vi "Zmienne funkcjonalne.vi"() -> ()   [LabVIEW 2020]
uses:
  Control 4.ctl
panel:
  out "XY Graph":cluster{"Array 2":dbl[], "Array 2":dbl[]}(graph)
  in  "Enum":T1
  out "Array":dbl[][](array[numeric])
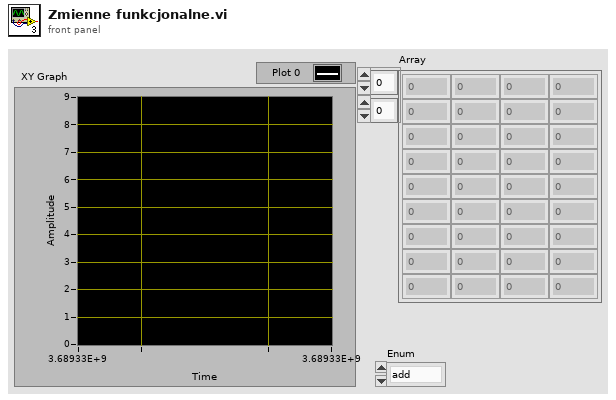
[diagram p1: front panel]
types:
  T1 = typedef "Control 4.ctl" = enum16{"add", "read", "readAll", "reset", "zapis_do_pliku", "odczyt_z_pliku"}
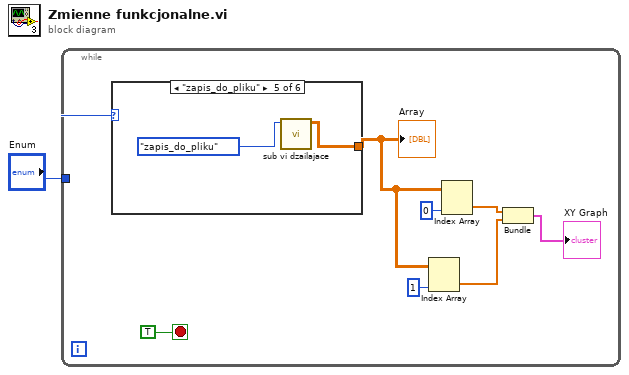
[diagram p0: block diagram]
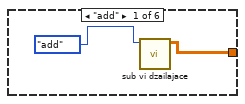
[diagram p2: hidden frame]
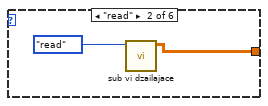
[diagram p3: hidden frame]
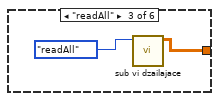
[diagram p4: hidden frame]
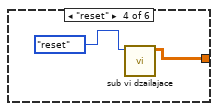
[diagram p5: hidden frame]
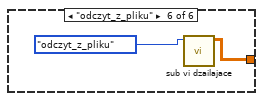
[diagram p6: hidden frame]
diagram:
  n1 = while {
    tunnel: "Enum" -> [w8]
    stop <- TRUE stop-if-true
    n2 = case shown="\"zapis_do_pliku\"" w8 {
      tunnel: [w10 w12 w14 w16 w18 w20] -> w5
      frame "add" {
        n3 = call "sub vi dzailajace.vi"("Enum in"=Control_4."add" ("Enum")) -> ("Array 2"=w10:dbl[][])  [unwired: 10 in]
      }
      frame "read" {
        n4 = call "sub vi dzailajace.vi"("Enum in"=Control_4."read" ("Enum")) -> ("Array 2"=w12:dbl[][])  [unwired: 10 in]
      }
      frame "readAll" {
        n5 = call "sub vi dzailajace.vi"("Enum in"=Control_4."readAll" ("Enum")) -> ("Array 2"=w14:dbl[][])  [unwired: 10 in]
      }
      frame "reset" {
        n6 = call "sub vi dzailajace.vi"("Enum in"=Control_4."reset" ("Enum")) -> ("Array 2"=w16:dbl[][])  [unwired: 10 in]
      }
      frame "zapis_do_pliku" {
        n7 = call "sub vi dzailajace.vi"("Enum in"=Control_4."zapis_do_pliku" ("Enum")) -> ("Array 2"=w18:dbl[][])  [unwired: 10 in]
      }
      frame "odczyt_z_pliku" {
        n8 = call "sub vi dzailajace.vi"("Enum in"=Control_4."odczyt_z_pliku" ("Enum")) -> ("Array 2"=w20:dbl[][])  [unwired: 10 in]
      }
    }
    "Array" <- w5
    n9 = Index Array(array=w5, index (col)=1) -> (element=w3:dbl[])  [unwired: 1 in]
    n10 = Index Array(array=w5, index (col)=0 ("disabled index (col)")) -> (element=w2:dbl[])  [unwired: 1 in]
    n11 = Bundle("Array 2"=w2, "Array 2"=w3) -> (→"XY Graph":cluster{"Array 2":dbl[], "Array 2":dbl[]})  [unwired: 1 in]
  }
